vi "lab1_example_sine_signal_generator.vi"() -> ()   [LabVIEW 2014]
uses:
  <vilib>/measure/maspectr.llb/Power Spectrum and PSD Export Mode.ctl
  <vilib>/Analysis/1siggen.llb/Ramp Pattern by Samples.vi
  sub_var_stop.vi
  <instrlib>/niUSRP/niUSRP Fetch Rx Data (CDB Cluster).vi
  <vilib>/measure/maspectr.llb/FFT Power Spectrum and PSD for 1 Chan (CDB).vi
  <instrlib>/niUSRP/niUSRP Write Tx Data (CDB Cluster).vi
  <vilib>/Analysis/NI_AALBase.lvlib
  <vilib>/measure/NI_MAPro.lvlib
panel:
  in  "gain 2":dbl format="%#_6f"
  in  "gain":dbl format="%#_6f"
  in  "device names 2":refnum<k15>
  in  "device names":refnum<k15>
  in  "number of samples":i64=20000
  out "coerced gain":dbl format="%#_6f"
  out "coerced carrier frequency":dbl=915000000.0 format="%#_6p"
  out "coerced IQ rate":dbl=200000.0 format="%#_6p"
  in  "carrier frequency":dbl=915000000.0 format="%#_6p"
  in  "IQ rate":dbl=200000.0 format="%#_6p"
  out "Waveform Graph 2":cluster{"f0":dbl, "df":dbl, "magnitude":dbl[]}(graph)
  out "Sine Wave":dbl[](graph)
  in  "duration":dbl format="%#_13g"
  in  "frequency":dbl format="%#_13g"
  in  "stop":bool
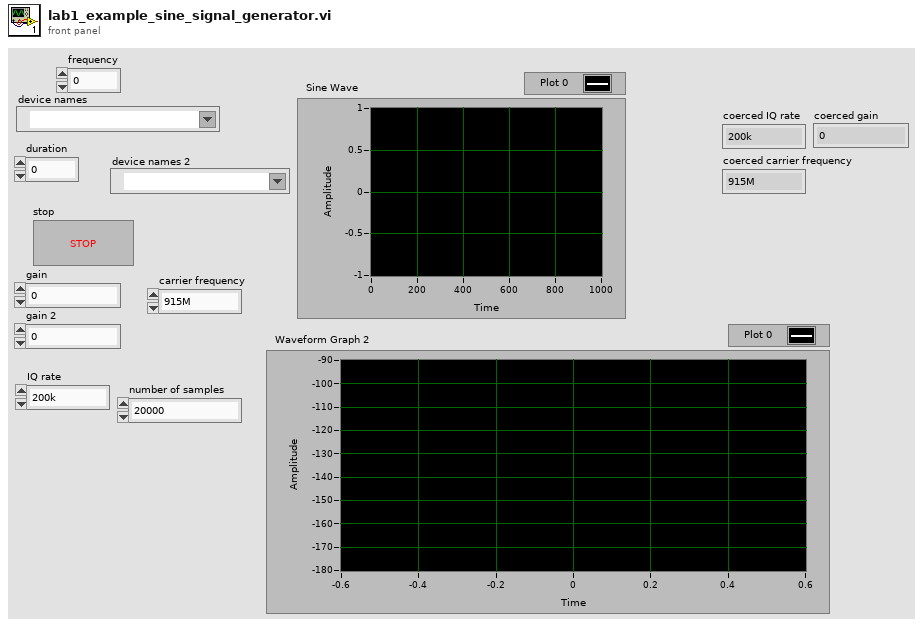
[diagram p1: front panel]
types:
  T1 = typedef "NI_MAPro.lvlib/Power Spectrum and PSD Export Mode.ctl" = u16
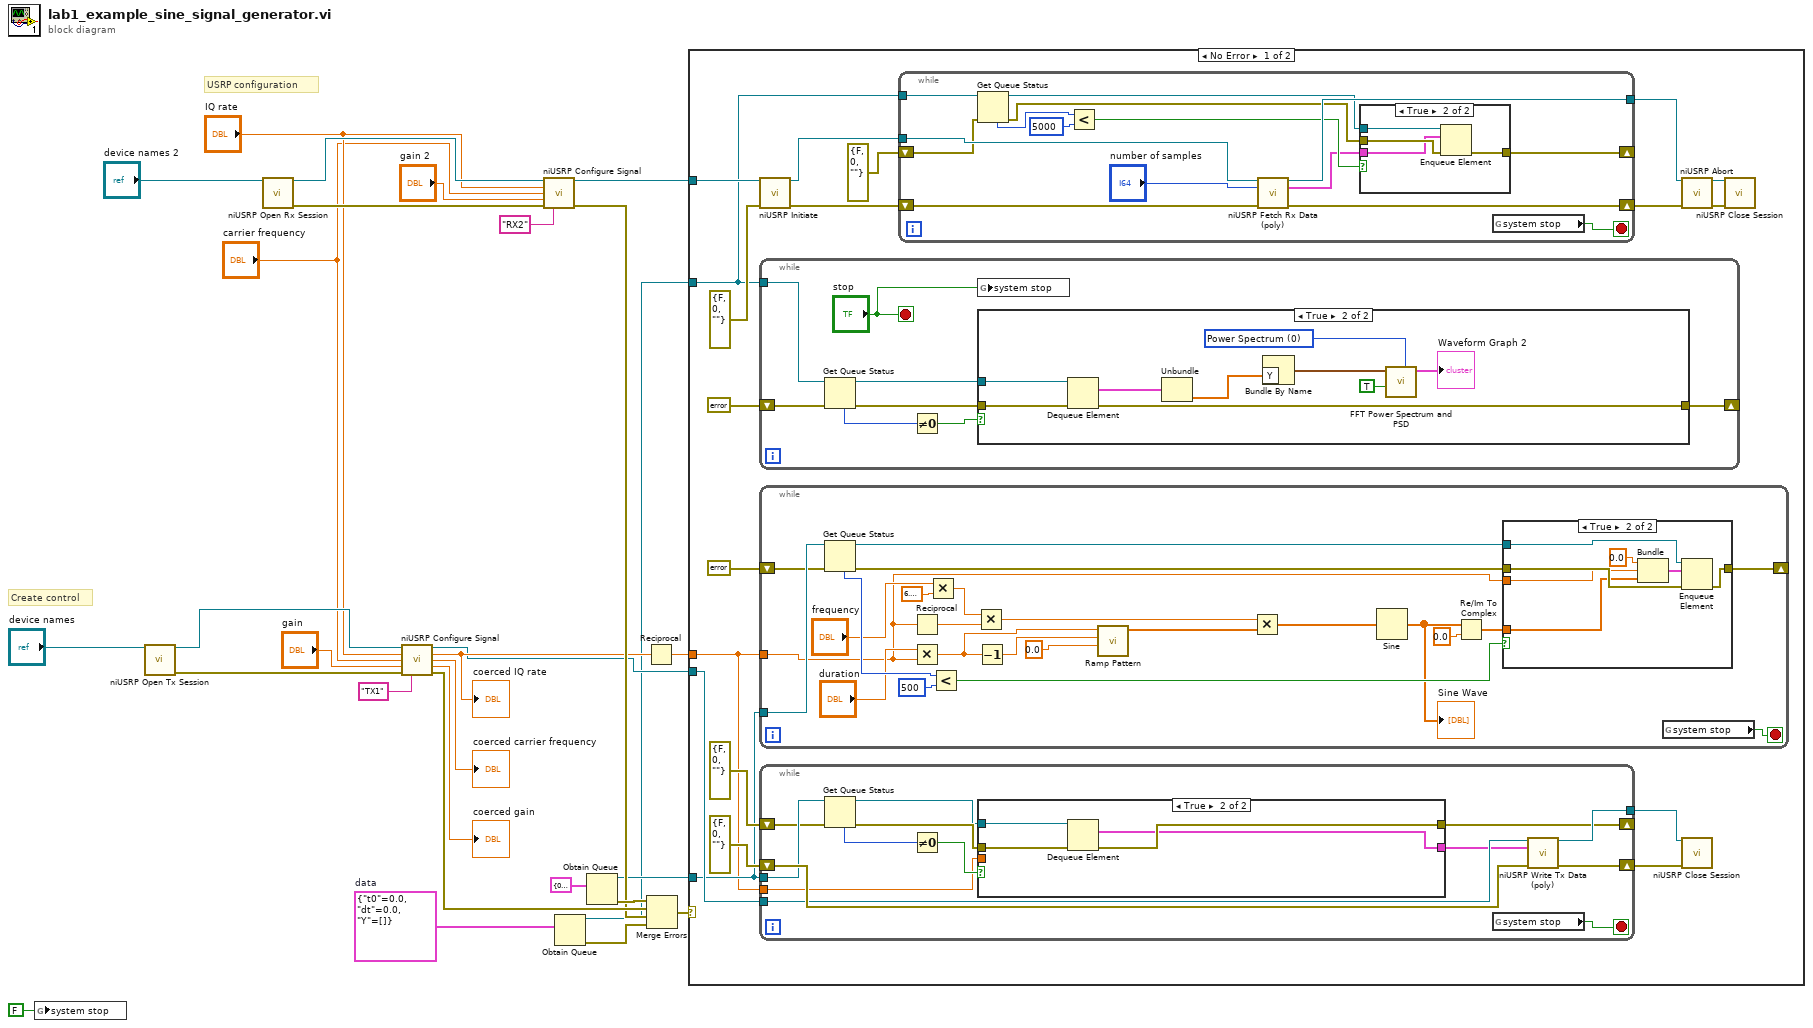
[diagram p0: block diagram]
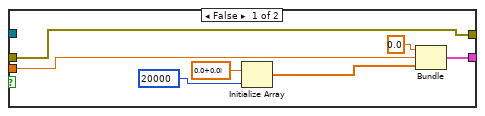
[diagram p3: hidden frame]
diagram:
  w15 = cluster{"t0":dbl, "dt":dbl, "Y":cdb[]} {"t0"=0.0, "dt"=0.0, "Y"=[]}  # data
  # "Create control"
  # "USRP configuration"
  n1 = global write "sub_var_stop.vi" "system stop"(FALSE) -> ()
  n2 = call <instrlib>:"niUSRP Open Tx Session.vi"("device names"="device names") -> ("session handle out"=w27:refnum<k15>, "error out"=w26:errorcluster)  [unwired: 13 in]
  n3 = call <instrlib>:"niUSRP Open Rx Session.vi"("device names"="device names 2") -> ("session handle out"=w25:refnum<k15>, "error out"=w24:errorcluster)  [unwired: 13 in]
  n4 = call <instrlib>:"niUSRP Configure Signal.vi"("session handle"=w27, "IQ rate"="IQ rate", "carrier frequency"="carrier frequency", "gain"="gain", "error in (no error)"=w26, "active antenna"="TX1") -> ("session handle out"=w9:refnum<k15>, "coerced IQ rate"=w12:dbl, "coerced carrier frequency"=→"coerced carrier frequency":dbl, "coerced gain"=→"coerced gain":dbl, "error out"=w18:errorcluster)  [unwired: 5 in]
  "coerced IQ rate" <- w12
  n5 = call <instrlib>:"niUSRP Configure Signal.vi"("session handle"=w25, "IQ rate"="IQ rate", "carrier frequency"="carrier frequency", "gain"="gain 2", "error in (no error)"=w24, "active antenna"="RX2") -> ("session handle out"=w5:refnum<k15>, "error out"=w17:errorcluster)  [unwired: 5 in, 3 out]
  n6 = Obtain Queue(element data type=w15) -> (queue out=w6:refnum<queue>, error out=w14:errorcluster)  [unwired: 4 in, 1 out]
  n7 = Obtain Queue(element data type=cluster{"t0":dbl, "dt":dbl, "Y":cdb[]} {"t0"=0.0, "dt"=1.0, "Y"=[]} ("data")) -> (queue out=w10:refnum<queue>, error out=w19:errorcluster)  [unwired: 4 in, 1 out]
  n8 = Reciprocal(x=w12) -> (1/x=w8:dbl)
  n9 = Merge Errors(w19, w18, w17, w14) -> (w7:errorcluster)
  n10 = case shown="No Error" w7 {
    tunnel: w10 -> [w40 _]
    tunnel: w9 -> [w41 _]
    tunnel: w8 -> [w39 _]
    tunnel: w6 -> [w29 _]
    tunnel: w5 -> [w30 _]
    frame No Error {
      n11 = call <instrlib>:"niUSRP Initiate.vi"("session handle"=w30, "error in (no error)"=errorcluster {"status"=FALSE, "code"=0, "source"=""}) -> ("session handle out"=w33:refnum<k15>, "error out"=w34:errorcluster)  [unwired: 12 in]
      n12 = while {
        tunnel: w29 -> [w99]
        shift-right: [w93] -> _
        shift-left: errorcluster {"status"=FALSE, "code"=0, "source"=""} ("error out") -> [w98]
        stop <- "stop" stop-if-true
        n13 = Get Queue Status(queue=w99, error in (no error)=w98) -> (queue out=w95:refnum<queue>, error out=w94:errorcluster, # elements in queue=w97:i32)  [unwired: 1 in, 5 out]
        n14 = Not Equal To 0?(x=w97) -> (x != 0?=w96:bool)
        n15 = global write "sub_var_stop.vi" "system stop"("stop") -> ()
        n16 = case shown="True" w96 {
          tunnel: w95 -> [_ w110]
          tunnel: w94 -> [w101 w109]
          tunnel: [w101 w108] -> w93
          frame False {
          }
          frame True {
            w104 = T1 0 items=["Power Spectrum", "Power Spectral Density"] ("export mode")
            n17 = Dequeue Element(queue=w110, error in (no error)=w109) -> (element=w103:cluster{"t0":dbl, "dt":dbl, "Y":cdb[]}, error out=w108:errorcluster)  [unwired: 1 in, 2 out]
            n18 = Unbundle "Unbundle"(w103) -> ("Y"=w102:cdb[])  [unwired: 2 out]
            n19 = Bundle By Name("Y"=w102) -> (w107:waveform(cdb))  [unwired: 1 in]
            n20 = call-poly <vilib>:"FFT Power Spectrum and PSD.vi"("export mode"=w104, "dB On (F)"=TRUE, "time signal"=w107) -> ("Power Spectrum / PSD"=→"Waveform Graph 2":cluster{"f0":dbl, "df":dbl, "magnitude":dbl[]})  [unwired: 5 in, 3 out]
          }
        }
      }
      n21 = while {
        tunnel: w40 -> [w130]
        shift-right: [w128] -> _
        shift-left: errorcluster {"status"=FALSE, "code"=0, "source"=""} ("error out") -> [w126]
        tunnel: w39 -> [w111]
        stop <- w134 stop-if-true
        n22 = Get Queue Status(queue=w130, error in (no error)=w126) -> (queue out=w129:refnum<queue>, error out=w127:errorcluster, # elements in queue=w125:i32)  [unwired: 1 in, 5 out]
        n23 = Reciprocal(x=w111) -> (1/x=w118:dbl)
        n24 = Multiply(x="duration", y=w111) -> (x*y=w116:dbl)
        n25 = Multiply(x="frequency", y=6.283185307179586) -> (x*y=w120:dbl)
        n26 = Less?(x=w125, y=500) -> (x < y?=w123:bool)
        n27 = Multiply(x=w120, y=w118) -> (x*y=w119:dbl)
        n28 = Decrement(x=w116) -> (x-1=w132:dbl)
        n29 = call-poly <vilib>:"Ramp Pattern.vi"("start"=0.0, "end"=w132, "samples"=w116) -> ("Ramp Pattern"=w131:dbl[])  [unwired: 7 in, 1 out]
        n30 = Multiply(x=w119, y=w131) -> (x*y=w115:dbl[])
        n31 = Sine(x=w115) -> (sin(x)=w113:dbl[])
        "Sine Wave" <- w113
        n32 = Re/Im To Complex(1:0.0 ("start"), 2:w113) -> (0:w112:cdb[])
        n33 = case shown="True" w123 {
          tunnel: w129 -> [_ w142]
          tunnel: [w135 w141] -> w128
          tunnel: w127 -> [w135 w140]
          tunnel: w111 -> [_ w137]
          tunnel: w112 -> [_ w136]
          frame False {
          }
          frame True {
            n34 = Bundle("start"=0.0, w137, w136) -> (w138:cluster{"start":dbl, dbl, cdb[]})  [unwired: 1 in]
            n35 = Enqueue Element(queue=w142, element=w138, error in (no error)=w140) -> (error out=w141:errorcluster)  [unwired: 1 in, 2 out]
          }
        }
        n36 = global read "sub_var_stop.vi" "system stop"() -> (w134:bool)
      }
      n37 = while {
        shift-right: [w80] -> w45
        shift-left: errorcluster {"status"=FALSE, "code"=0, "source"=""} ("error out") -> [w78]
        tunnel: [w79] -> w44
        tunnel: w41 -> [w77]
        tunnel: w40 -> [w76]
        shift-right: [w71] -> _
        shift-left: errorcluster {"status"=FALSE, "code"=0, "source"=""} ("error out") -> [w75]
        tunnel: w39 -> [w68]
        stop <- w81 stop-if-true
        n38 = Get Queue Status(queue=w76, error in (no error)=w75) -> (queue out=w70:refnum<queue>, error out=w72:errorcluster, # elements in queue=w74:i32)  [unwired: 1 in, 5 out]
        n39 = Not Equal To 0?(x=w74) -> (x != 0?=w73:bool)
        n40 = case shown="True" w73 {
          tunnel: w72 -> [w83 w92]
          tunnel: [w83 w91] -> w71
          tunnel: w70 -> [_ w90]
          tunnel: [w88 w89] -> w69
          tunnel: w68 -> [w82 _]
          frame False {
            n41 = Initialize Array(cdb 0.0+0.0i, 20000 ("dimension size")) -> (w85:cdb[])
            n42 = Bundle(0.0, w82, w85) -> (w88:cluster{dbl, dbl, cdb[]})  [unwired: 1 in]
          }
          frame True {
            n43 = Dequeue Element(queue=w90, error in (no error)=w92) -> (element=w89:cluster{"t0":dbl, "dt":dbl, "Y":cdb[]}, error out=w91:errorcluster)  [unwired: 1 in, 2 out]
          }
        }
        n44 = global read "sub_var_stop.vi" "system stop"() -> (w81:bool)
        n45 = call-poly <instrlib>:"niUSRP Write Tx Data (poly).vi"("session handle"=w77, "data"=w69, "error in (no error)"=w78) -> ("session handle out"=w79:refnum<k15>, "error out"=w80:errorcluster)  [unwired: 11 in]
      }
      n46 = while {
        tunnel: w33 -> [w61]
        shift-right: [w57] -> w35
        shift-left: w34 -> [w60]
        tunnel: [w58] -> w36
        tunnel: w29 -> [w56]
        shift-right: [w48] -> _
        shift-left: errorcluster {"status"=FALSE, "code"=0, "source"=""} ("error out") -> [w55]
        stop <- w62 stop-if-true
        n47 = Get Queue Status(queue=w56, error in (no error)=w55) -> (queue out=w51:refnum<queue>, error out=w50:errorcluster, # elements in queue=w54:i32)  [unwired: 1 in, 5 out]
        n48 = Less?(x=w54, y=5000) -> (x < y?=w52:bool)
        n49 = call-poly <instrlib>:"niUSRP Fetch Rx Data (poly).vi"("session handle"=w61, "number of samples"="number of samples", "error in (no error)"=w60) -> ("session handle out"=w58:refnum<k15>, "data"=w49:cluster{"t0":dbl, "dt":dbl, "Y":cdb[]}, "error out"=w57:errorcluster)  [unwired: 9 in, 1 out]
        n50 = case shown="True" w52 {
          tunnel: w51 -> [_ w67]
          tunnel: w50 -> [w63 w66]
          tunnel: w49 -> [_ w65]
          tunnel: [w63 w64] -> w48
          frame False {
          }
          frame True {
            n51 = Enqueue Element(queue=w67, element=w65, error in (no error)=w66) -> (error out=w64:errorcluster)  [unwired: 1 in, 2 out]
          }
        }
        n52 = global read "sub_var_stop.vi" "system stop"() -> (w62:bool)
      }
      n53 = call <instrlib>:"niUSRP Abort.vi"("session handle"=w36, "error in (no error)"=w35) -> ("session handle out"=w31:refnum<k15>, "error out"=w32:errorcluster)  [unwired: 12 in]
      n54 = call <instrlib>:"niUSRP Close Session.vi"("session handle"=w44, "error in (no error)"=w45) -> ()  [unwired: 13 in, 1 out]
      n55 = call <instrlib>:"niUSRP Close Session.vi"("session handle"=w31, "error in (no error)"=w32) -> ()  [unwired: 13 in, 1 out]
    }
    frame Error {
    }
  }
